vi "String to sensor value.vi"(11 "String":string) -> (3 "Numeric":dbl)   [LabVIEW 2020, in "Arduino-Adafruit stepper.lvlib"]
uses:
  Arduino-Adafruit stepper.lvlib
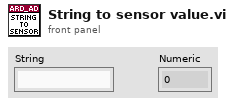
[diagram p1: front panel]
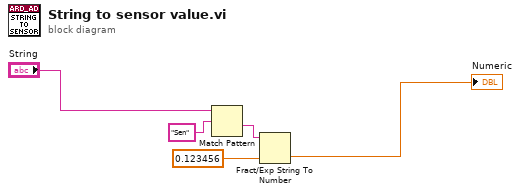
[diagram p0: block diagram]
diagram:
  n1 = Match Pattern(string="String", regular expression="Sen") -> (after substring=w3:string)  [unwired: 1 in, 3 out]
  n2 = Fract/Exp String To Number(string=w3, default (0 dbl)=0.123456 ("default (0 DBL)")) -> (number=→"Numeric":dbl)  [unwired: 2 in, 1 out]
